vi "changeState.vi"(8 "error in (no error)":errorcluster, 10 "State:":T1, 11 "Model in":refnum<class "Model.lvclass">) -> (0 "error out":errorcluster, 3 "Model out":refnum<class "Model.lvclass">)   [LabVIEW 2013, in "Model.lvclass"]
uses:
  Model.lvclass
  Typedefs/StateSelector.ctl
  Model.lvclass/Model.ctl
  ApplicationElements/Logger/Logger.lvclass/Logger.ctl
  ApplicationElements/Logger/Logger.lvclass
  Typedefs/M2AADTTypedefs.lvlib
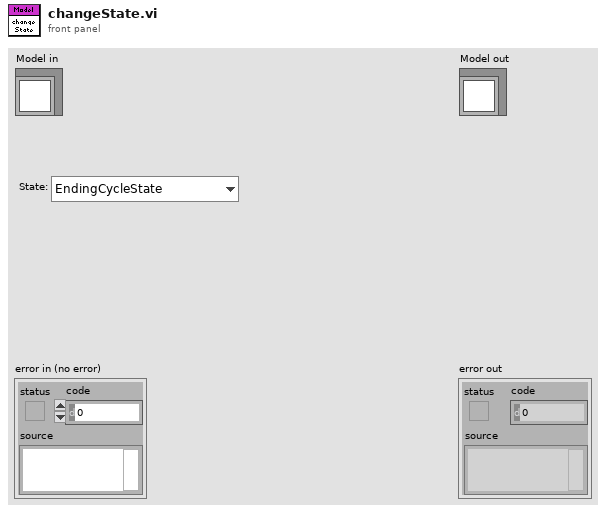
[diagram p1: front panel]
types:
  T1 = typedef "M2AADTTypedefs.lvlib/StateSelector.ctl" = enum16{"EndingCycleState", "FaultState", "InteractiveMotionState", "MovingToNewForceState", "OffState", "PausingState", "StandbyState", "StoppedState"}
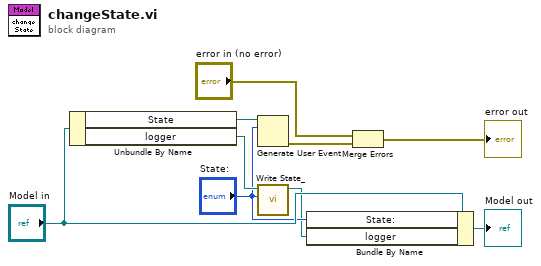
[diagram p0: block diagram]
diagram:
  n1 = Unbundle By Name("Model in") -> ("State"=w9:refnum<user-event>, "logger"=w3:refnum<class "Logger.lvclass">)
  n2 = Generate User Event(user event=w9, event data cluster="State:") -> (error out=w5:errorcluster)  [unwired: 2 in, 1 out]
  n3 = call "Write State_.vi"("State:"="State:", "Logger in"=w3) -> ("Logger out"=w1:refnum<class "Logger.lvclass">)  [unwired: 9 in]
  n4 = Bundle By Name(cluster="Model in", "State:"="State:", "logger"=w1) -> (→"Model out":refnum<class "Model.lvclass">)
  n5 = Merge Errors("error in (no error)", w5) -> (→"error out":errorcluster)
